vi "Send Move Stage.vi"(7 "Message Priority (Normal)":T1=enum."Normal", 8 "error in (no error)":errorcluster, 9 "Y Axis":dbl, 10 "X Axis":dbl, 11 "Interlock Q Class":refnum<class "Interlock Q Class.lvclass">) -> (0 "error out":errorcluster, 3 "Interlock Q Class":refnum<class "Interlock Q Class.lvclass">)   [LabVIEW 2022 SP3, in "XY Stage Process.lvlib" / "Move Stage Msg.lvclass"]
doc: "This VI sends the message to an actor."
uses:
  Move Stage Msg.lvclass
  <vilib>/ActorFramework/Message Enqueuer/Message Priority.ctl
  C:/Program Files/National Instruments/LabVIEW 2022/vi.lib/ActorFramework/Message/Message.lvclass
  Move Stage Msg.lvclass/Move Stage Msg.ctl
  <vilib>/ActorFramework/Message Enqueuer/Message Enqueuer.lvclass/Message Enqueuer.ctl
  <vilib>/ActorFramework/Message Priority Queue/Priority Enqueue.vi
  Interlock Q Class/Interlock Q Class.lvclass
  C:/Stage-Work/MAS/XY Stage Process/XY Stage Process/XY Stage Process Messages/Move Stage Msg/Move Stage Msg.lvclass
  <vilib>/ActorFramework/Message Enqueuer/Message Enqueuer.lvclass
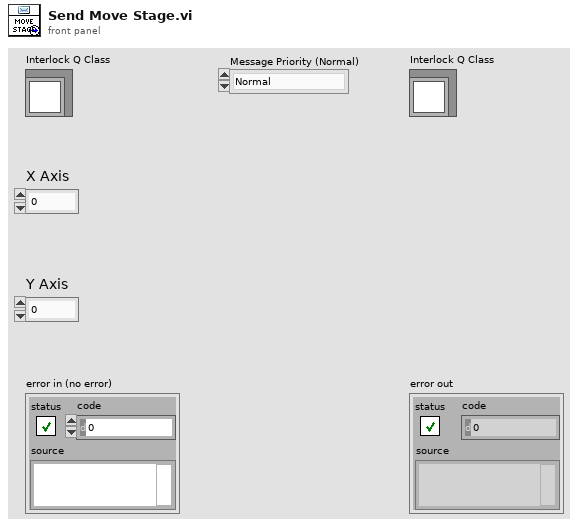
[diagram p1: front panel]
types:
  T1 = typedef "Actor Framework.lvlib/Message Enqueuer.lvclass/Message Priority.ctl" = enum16{"Low", "Normal", "High"}
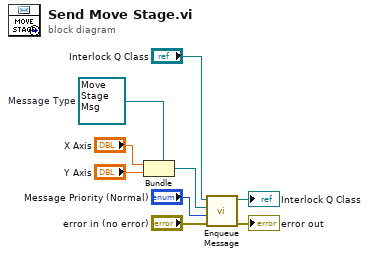
[diagram p0: block diagram]
diagram:
  w9 = refnum<class "Move Stage Msg.lvclass"> refnum  # Message Type
  n1 = Bundle(cluster=w9, "X Axis", "Y Axis") -> (w6:refnum<class "Move Stage Msg.lvclass">)
  n2 = call-dynamic "Enqueue Message.vi"("error in (no error)"="error in (no error)", "Message Priority (Normal)"="Message Priority (Normal)", "Message"=w6, "Interlock Q Class in"="Interlock Q Class") -> ("error out"=→"error out":errorcluster, "Interlock Q Class out"=→"Interlock Q Class":refnum<class "Interlock Q Class.lvclass">)  [unwired: 6 in]
